vi "Impedance Correction.vi"() -> ()   [LabVIEW 2024]
uses:
  <vilib>/Utility/file.llb/Read From Spreadsheet File (DBL).vi
  <vilib>/Utility/file.llb/Write Delimited Spreadsheet (DBL).vi
  260f672a-c3a2-44e7-8212-110ef4c2a241.vi
  d023b0aa-14ab-49f5-9e90-6c0e408ecbac.vi
panel:
  in  "Current Channels":string[](array[string])=["I X1 (Resampled)", "I Y1 (Resampled)"]
  in  "X channel":string="Field_fixed (Resampled)"
  in  "Group":string="p"
  in  "Signal Channels":string[](array[string])=["Vc1 X1 (Resampled)", "Vc1 Y1 (Resampled)"]
  in  "Save Button":bool
  in  "Chan #":i32=-1
  out "Current":cluster{"all rows":dbl[], dbl[]}[](graph)
  in  "Divide by current chan #":i32=-1
  in  "Fequency":dbl=300000.0 format="%#_6p"
  in  "stop":bool
  in  "V -> Impedance factor":dbl=100.0
  in  "C (parallel)":dbl(slide)=1e-09 step=1e-11 scale=0.0..5e-08 scale format="%#_6p"
  in  "L (series)":dbl(slide)=1e-15 scale=0.0..1e-12 scale format="%#_6p"
  in  "Phase":dbl(slide) step=0.1 scale=-180.0..180.0
  out "Data and Fix":cluster{"all rows":dbl[], dbl[]}[](graph)
  in  "Input file path":path
  # "=R_mon*GainI/GainV\n= 1/Gain/current"
  # "Fix:  R=(I/V-Z_C^-1)^-1-Z_L"
  # "Z=((R+ZL)^?-1+ZC^-1))^-1\nV=I*Z\nV/I=((R+ZL)^-1+ZC^-1))^-1\nI/V=(R+ZL)^-1+ZC^-1\n(I/V-ZC^-1)^-1-ZL=R"
  # "Column_X=chan # *2 +1\nColumn_Y=Column_X+1"
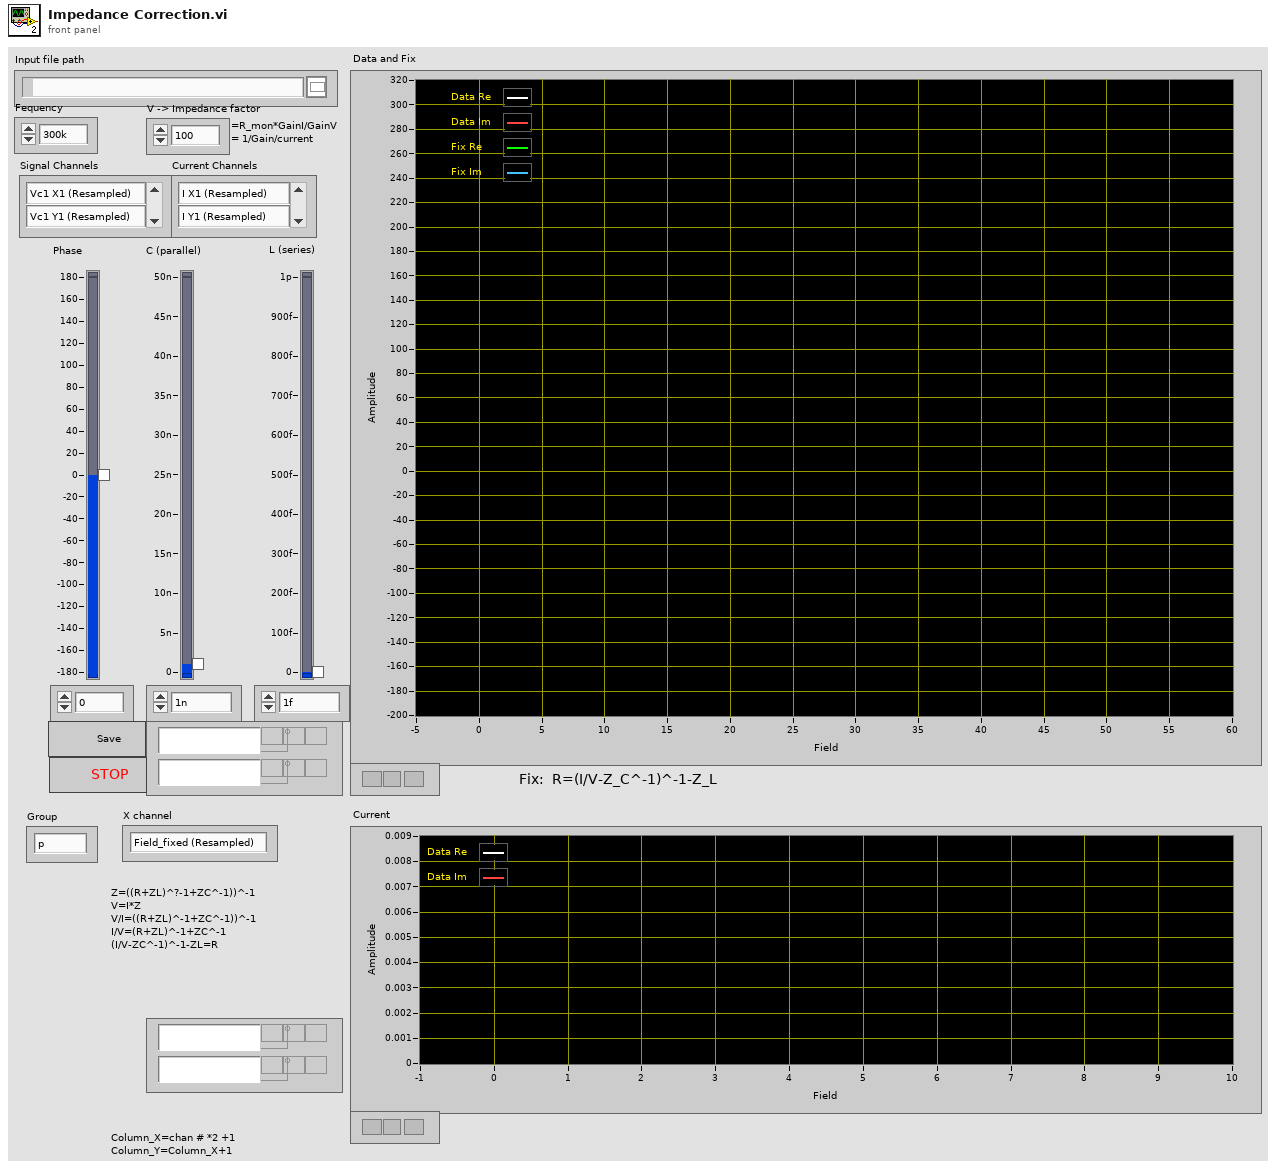
[diagram p1: front panel]
types:
  T1 = enum16{"open", "open or create", "create or replace", "create", "open (read-only)"}
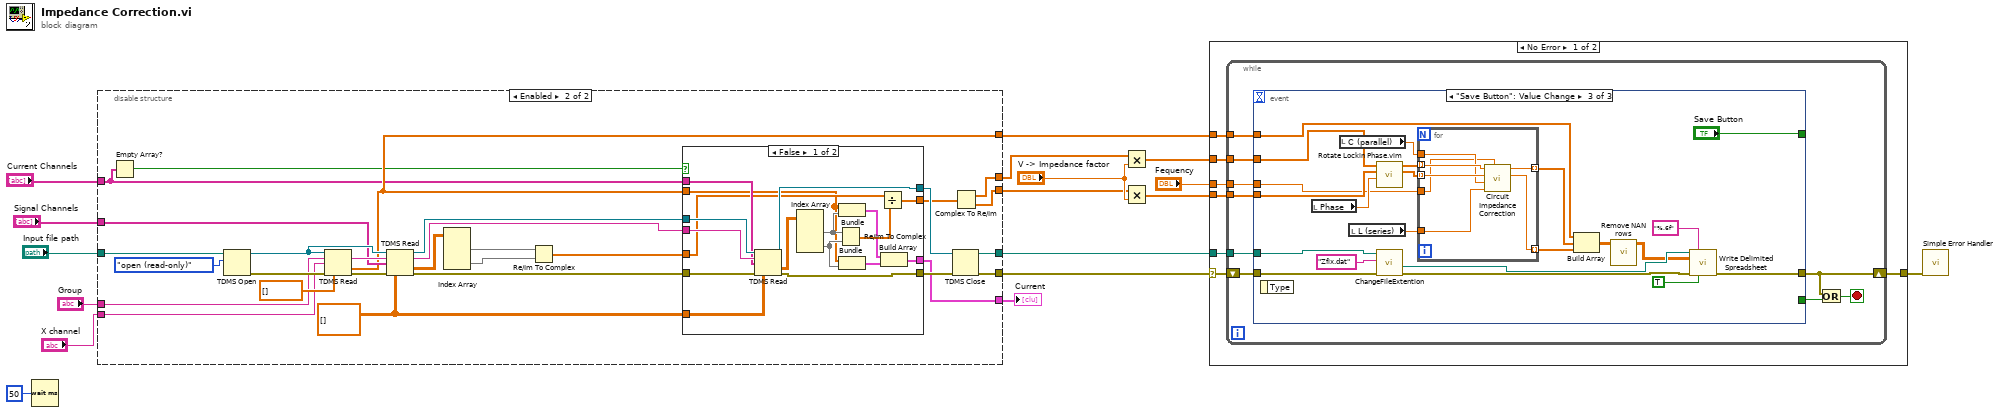
[diagram p0: block diagram]
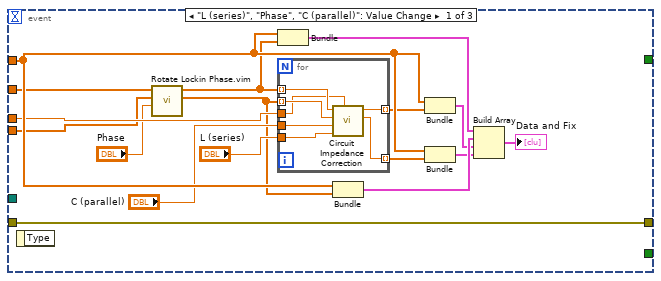
[diagram p2: hidden frame]
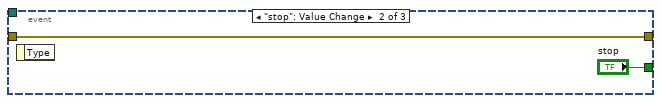
[diagram p3: hidden frame]
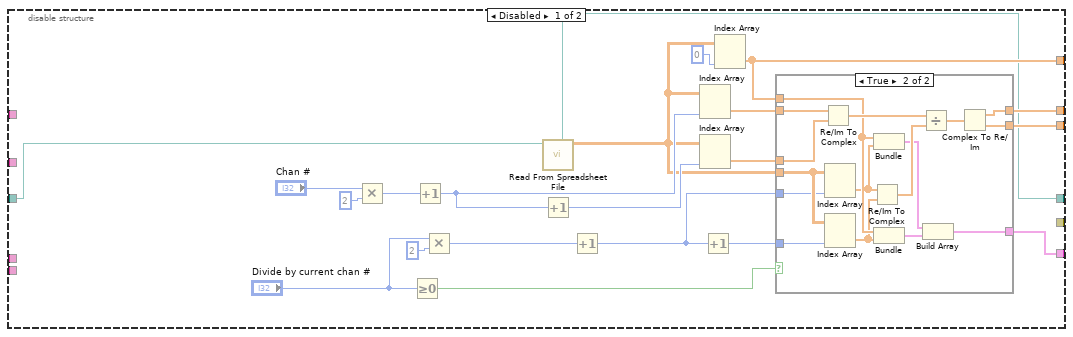
[diagram p5: hidden frame]
diagram:
  n1 = Wait (ms)(milliseconds to wait=u32 50) -> ()  [unwired: 1 out]
  n2 = disable-structure shown="Enabled" {
    disable-tunnel: [w36 w61] -> w13
    disable-tunnel: [w34 w60] -> w12
    disable-tunnel: [w27 w63] -> w11
    disable-tunnel: "Input file path" -> [w21 w76]
    disable-tunnel: [w19 w70] -> w8
    disable-tunnel: "Group" -> [_ w75]
    disable-tunnel: "X channel" -> [_ w74]
    disable-tunnel: "Signal Channels" -> [_ w73]
    disable-tunnel: "Current Channels" -> [_ w58]
    disable-tunnel: [w18 w62] -> w3
    disable-tunnel: [_ w59] -> w1
    frame Disabled {
      n3 = Multiply(x="Chan #", y=2) -> (x*y=w26:i32)
      n4 = Greater Or Equal To 0?(x="Divide by current chan #") -> (x >= 0?=w28:bool)
      n5 = Increment(x=w26) -> (x+1=w24:i32)
      n6 = Multiply(x="Divide by current chan #", y=2) -> (x*y=w31:i32)
      n7 = call-poly <vilib>:"Read From Spreadsheet File.vi"("file path (dialog if empty)"=w21) -> ("all rows"=w20:dbl[][], "new file path (Not A Path if cancelled)"=w19:path)  [unwired: 6 in, 3 out]
      n8 = Increment(x=w24) -> (x+1=w23:i32)
      n9 = Increment(x=w31) -> (x+1=w30:i32)
      n10 = Index Array(array=w20, index (col)=w24) -> (element=w37:dbl[])  [unwired: 1 in]
      n11 = Index Array(array=w20, index (col)=w23) -> (element=w35:dbl[])  [unwired: 1 in]
      n12 = Increment(x=w30) -> (x+1=w29:i32)
      n13 = Index Array(array=w20, index (col)=0 ("disabled index (col)")) -> (element=w27:dbl[])  [unwired: 1 in]
      n14 = case shown="True" w28 {
        tunnel: w37 -> [w40 w53]
        tunnel: [w40 w48] -> w36
        tunnel: w35 -> [w39 w52]
        tunnel: [w39 w47] -> w34
        tunnel: w20 -> [_ w56]
        tunnel: w30 -> [_ w55]
        tunnel: w29 -> [_ w54]
        tunnel: w27 -> [_ w44]
        tunnel: [_ w41] -> w18
        frame False {
        }
        frame True {
          n15 = Re/Im To Complex(1:w52, 2:w53) -> (0:w51:cdb[])
          n16 = Index Array(array=w56, index (col)=w55) -> (element=w43:dbl[])  [unwired: 1 in]
          n17 = Index Array(array=w56, index (col)=w54) -> (element=w42:dbl[])  [unwired: 1 in]
          n18 = Re/Im To Complex(1:w42, 2:w43) -> (0:w50:cdb[])
          n19 = Bundle("all rows"=w44, "all rows"=w43) -> (w46:cluster{"all rows":dbl[], "all rows":dbl[]})  [unwired: 1 in]
          n20 = Bundle("all rows"=w44, "all rows"=w42) -> (w45:cluster{"all rows":dbl[], "all rows":dbl[]})  [unwired: 1 in]
          n21 = Divide(x=w51, y=w50) -> (x/y=w49:cdb[])
          n22 = Build Array(w46, w45) -> (w41:cluster{"all rows":dbl[], "all rows":dbl[]}[])
          n23 = Complex To Re/Im(x + iy=w49) -> (x=w48:dbl[], y=w47:dbl[])
        }
      }
    }
    frame Enabled {
      w64 = dbl[][] [] ("all rows")
      n24 = Empty Array?(array=w58) -> (empty?=w57:bool)
      n25 = TDMS Open(10:T1."open (read-only)" ("operation (0:open)"), 11:w76) -> (0:w81:errorcluster, 3:w83:refnum<k34>)  [unwired: 5 in]
      n26 = TDMS Read(0:w83, 5:w75, 7:w74, 11:w81, 12:dbl[] [] ("all rows")) -> (6:w84:string, 10:w63:dbl[], 15:w82:errorcluster)  [unwired: 3 in, 3 out]
      n27 = TDMS Read(0:w83, 5:w84, 7:w73, 11:w82, 12:w64) -> (4:w78:refnum<k34>, 6:w80:string, 10:w67:dbl[][], 15:w79:errorcluster)  [unwired: 3 in, 2 out]
      n28 = Index Array(array=w67) -> (element #1=w66:dbl[], element #2=w65:dbl[])  [unwired: 4 in]
      n29 = Re/Im To Complex(1:w65, 2:w66) -> (0:w69:cdb[])
      n30 = case shown="False" w57 {
        tunnel: w80 -> [w102 _]
        tunnel: w79 -> [w101 w105]
        tunnel: w78 -> [w100 w104]
        tunnel: w58 -> [w99 _]
        tunnel: [w98 w105] -> w72
        tunnel: [w97 w104] -> w71
        tunnel: w69 -> [w96 w103]
        tunnel: [w94 w103] -> w68
        tunnel: w64 -> [w91 _]
        tunnel: w63 -> [w87 _]
        tunnel: [w86 _] -> w62
        frame False {
          n31 = TDMS Read(0:w100, 5:w102, 7:w99, 11:w101, 12:w91) -> (4:w97:refnum<k34>, 10:w90:dbl[][], 15:w98:errorcluster)  [unwired: 3 in, 3 out]
          n32 = Index Array(array=w90) -> (element #1=w88:dbl[], element #2=w89:dbl[])  [unwired: 4 in]
          n33 = Re/Im To Complex(1:w89, 2:w88) -> (0:w95:cdb[])
          n34 = Bundle("all rows"=w87, "all rows"=w88) -> (w93:cluster{"all rows":dbl[], "all rows":dbl[]})  [unwired: 1 in]
          n35 = Bundle("all rows"=w87, "all rows"=w89) -> (w92:cluster{"all rows":dbl[], "all rows":dbl[]})  [unwired: 1 in]
          n36 = Divide(x=w96, y=w95) -> (x/y=w94:cdb[])
          n37 = Build Array(w93, w92) -> (w86:cluster{"all rows":dbl[], "all rows":dbl[]}[])
        }
        frame True {
        }
      }
      n38 = TDMS Close(8:w72, 11:w71) -> (0:w59:errorcluster, 3:w70:path)
      n39 = Complex To Re/Im(x + iy=w68) -> (x=w61:dbl[], y=w60:dbl[])
    }
  }
  "Current" <- w3
  n40 = Multiply(x=w13, y="V -> Impedance factor") -> (x*y=w17:dbl[])
  n41 = Multiply(x=w12, y="V -> Impedance factor") -> (x*y=w16:dbl[])
  n42 = case shown="No Error" w1 {
    selector: w1 -> [w106 w177]
    tunnel: w17 -> [w112 _]
    tunnel: w16 -> [w111 _]
    tunnel: "Fequency" -> [w110 _]
    tunnel: w11 -> [w109 _]
    tunnel: w8 -> [w108 _]
    tunnel: [w107 w177] -> w2
    frame No Error {
      n43 = while {
        tunnel: w112 -> [w118]
        tunnel: w111 -> [w117]
        tunnel: w109 -> [w121]
        tunnel: w110 -> [w119]
        tunnel: w108 -> [w116]
        shift-right: [w113] -> w107
        shift-left: w106 -> [w115]
        stop <- w114 stop-if-true
        n44 = event shown="[2] \"Save Button\": Value Change" {
          selector: _ -> [_ _ _]
          dyn-events: _ -> [_ _ _]
          timeout: _ -> [_ _ _]
          tunnel: w121 -> [w138 _ w158]
          tunnel: [_ "stop" _] -> w120
          tunnel: w119 -> [w134 _ w161]
          tunnel: w118 -> [w126 _ w165]
          tunnel: w117 -> [w124 _ w164]
          tunnel: [_ _ "Save Button"] -> _
          tunnel: w116 -> [_ _ w159]
          tunnel: w115 -> [w122 w146 w150]
          tunnel: [w122 w146 w148] -> w113
          event "L (series)", "Phase", "C (parallel)": Value Change {
            n45 = event-data() -> ()  [unwired: 1 in, 1 out]
            n46 = call "Rotate Lockin Phase.vim"("Phase"="Phase", "Array Y in"=w124, "Array X in"=w126) -> ("Array Y out"=w123:dbl[], "Array X out"=w125:dbl[])  [unwired: 7 in]
            n47 = Bundle("all rows"=w138, "Array X out"=w125) -> (w137:cluster{"all rows":dbl[], "Array X out":dbl[]})  [unwired: 1 in]
            n48 = for {
              tunnel: w125 -> [w145] mode=indexing
              tunnel: w123 -> [w144] mode=indexing
              tunnel: "C (parallel)" -> [w143]
              tunnel: w134 -> [w142]
              tunnel: "L (series)" -> [w141]
              tunnel: [w140] -> w132 mode=indexing
              tunnel: [w139] -> w131 mode=indexing
              n49 = call "Circuit Impedance Correction.vi"("Fequency"=w142, "Series inductance"=w141, "Parallel capacitance"=w143, "Measured Resistance Y"=w144, "Measured Resistance X"=w145) -> ("Corrected resistance Y"=w139:dbl, "Corrected resistance X"=w140:dbl)  [unwired: 4 in, 1 out]
            }
            n50 = Bundle("all rows"=w138, "Array Y out"=w123) -> (w136:cluster{"all rows":dbl[], "Array Y out":dbl[]})  [unwired: 1 in]
            n51 = Bundle("all rows"=w138, w132) -> (w130:cluster{"all rows":dbl[], dbl[]})  [unwired: 1 in]
            n52 = Bundle("all rows"=w138, w131) -> (w129:cluster{"all rows":dbl[], dbl[]})  [unwired: 1 in]
            n53 = Build Array(w137, w136, w130, w129) -> (→"Data and Fix":cluster{"all rows":dbl[], "Array Y out":dbl[]}[])
          }
          event "stop": Value Change {
            n54 = event-data() -> ()  [unwired: 1 in, 1 out]
          }
          event "Save Button": Value Change {
            n55 = event-data() -> ()  [unwired: 1 in, 1 out]
            n56 = local read "Phase"() -> (w166:dbl)
            n57 = local read "C (parallel)"() -> (w162:dbl)
            n58 = local read "L (series)"() -> (w163:dbl)
            n59 = call "Rotate Lockin Phase.vim"("Phase"=w166, "Array Y in"=w164, "Array X in"=w165) -> ("Array Y out"=w167:dbl[], "Array X out"=w168:dbl[])  [unwired: 7 in]
            n60 = call "ChangeFileExtention.vi"("Error In"=w150, "New extension"="Zfix.dat" ("New Extention"), "File Path"=w159) -> ("Error Out"=w149:errorcluster, "Path with new extension"=w153:path)  [unwired: 1 in, 6 out]
            n61 = for {
              tunnel: w168 -> [w176] mode=indexing
              tunnel: w167 -> [w175] mode=indexing
              tunnel: w162 -> [w174]
              tunnel: w161 -> [w173]
              tunnel: w163 -> [w172]
              tunnel: [w171] -> w157 mode=indexing
              tunnel: [w170] -> w156 mode=indexing
              n62 = call "Circuit Impedance Correction.vi"("Fequency"=w173, "Series inductance"=w172, "Parallel capacitance"=w174, "Measured Resistance Y"=w175, "Measured Resistance X"=w176) -> ("Corrected resistance Y"=w170:dbl, "Corrected resistance X"=w171:dbl)  [unwired: 4 in, 1 out]
            }
            n63 = Build Array(w158, w157, w156) -> (w155:dbl[][])
            n64 = call "Remove NAN rows.vi"("Array - Numeric"=w155) -> ("Array out"=w152:dbl[][])  [unwired: 10 in]
            n65 = call-poly <vilib>:"Write Delimited Spreadsheet.vi"("file path (dialog if empty)"=w153, "format (%.3f)"="%.6f", "2D data"=w152, "error in (no error)"=w149, "transpose? (no:F)"=TRUE) -> ("error out"=w148:errorcluster)  [unwired: 9 in, 1 out]
          }
        }
        n66 = Or(x=w113, y=w120) -> (x .or. y?=w114:bool)
      }
    }
    frame Error {
    }
  }
  n67 = call <vilib>:"Simple Error Handler.vi"("error in (no error)"=w2) -> ()  [unwired: 4 in, 5 out]
